vi "MainGUI.vi"() -> ()   [LabVIEW 2017]
uses:
  General/Controls/Queue Manager Actions.ctl
  General/Controls/MessagePacket.ctl
  General/Controls/QueueNames.ctl
  General/Controls/FGV Actions.ctl
  Hardware/Main Scan Processor Status.vi
  Hardware/Table Stage/Controls/Motion Translation Module Control.ctl
  General/Controls/Set Get Controls.ctl
  General/Controls/ScanType.ctl
  General/Controls/Translation Stage Types.ctl
  Hardware/Table Stage/Controls/Translation Stage Cluster.ctl
  General/Controls/System Parameters.ctl
panel:
  in  "Status":string
  in  "Quit":bool
  in  "Scan Type":T1
  in  "Acquire":bool
  in  "Control Panel":enum32{"Scan", "Config", "Manual Contorls"}(tab)
  in  "Y":u16=1 min=1 max=30 step=1
  in  "X":u16=1 min=1 max=30 step=1
  in  "Custom":bool
  in  "XY Image Resolution":T2(ring)
  in  "C Frame Ave.":u8=1 min=1 max=30 step=1
  in  "B Frame Ave.":u8=1 min=1 max=30 step=1
  in  "Display Channel":T3(ring)
  in  "Zoom Factor":u8(knob)=1 min=1 max=10 step=1 scale=1.0..10.0
  in  "Pixel Dwell Time":dbl[unit] min=0.0 max=0.01 step=1e-05
  in  "A Frame Ave.":u8=1 min=1 max=30 step=1
  in  "Pockel Cell Delay":dbl[unit] min=0.0 max=0.01 step=1e-05
  in  "Galvo Setting Time":dbl[unit] min=0.0 max=0.01 step=1e-05
  in  "Max Line Rate":dbl[unit] min=0.0 max=10.0 step=0.01
  in  "Objective EFL":dbl[unit] min=0.0 max=0.01 step=1e-05
  in  "Angular Mag.":dbl min=0.0 max=10.0 step=0.01
  in  "Center Galvos":bool
  out "Label Name":string[][](array[string])
  in  "System Parameters":T4={"Optical /HW Parameters"={"Focal Length [mm]"=1.0, "Scan Lens EFL[mm]"=0.0, "Tube Lens EFL[mm]"=0.0, "Galvo V Range (+/-)"=0.0, "Galvo Max Half Angle [Deg]"=0.0, "Max Galvo Range[%]"=0.0}, "Vibratome"={"Z Bottom [mm]"=0.0, "Pre Cut Dwell [s]"=0.0, "Blade Frequency [RPM]"=0, "Slice Speed [mm/s]"=0.0, "Post Cut Dwell [s]"=0.0, "Ramp Time [s]"=0.0, "Start X [mm]"=0.0, "Start Y [mm]"=0.0, "Slice Length [mm]"=0.0, "Slice Axis"=enum."X Axis", "Controller VISA Ref"="COM4"}, "Table Stages"={"X Stage"={"Position"=0.0, "Is.Enabled?"=FALSE, "Is.Connected?"=FALSE, "Device SN"="45876539", "AccelerationMaximum"=0.0, "VelocityMaximum"=0.0, "Acceleration"=0.0, "Velocity"=0.0, "waitTimeout (ms)"=0, "Model"=enum."None", "Is.Homed?"=FALSE}, "Y Stage"={"Position"=0.0, "Is.Enabled?"=FALSE, "Is.Connected?"=FALSE, "Device SN"="45876539", "AccelerationMaximum"=0.0, "VelocityMaximum"=0.0, "Acceleration"=0.0, "Velocity"=0.0, "waitTimeout (ms)"=0, "Model"=enum."None", "Is.Homed?"=FALSE}, "Z Stage"={"Position"=0.0, "Is.Enabled?"=FALSE, "Is.Connected?"=FALSE, "Device SN"="45876539", "AccelerationMaximum"=0.0, "VelocityMaximum"=0.0, "Acceleration"=0.0, "Velocity"=0.0, "waitTimeout (ms)"=0, "Model"=enum."None", "Is.Homed?"=FALSE}}, "Imaging Parameter"={"Pixel Dwell Time [ms]"=1.0, "XY Center [um]"={"X"=1.0, "Y"=1.0}, "Zoom Factor"=1.0, "Display Channel"=enum."Channel A", "XY Image Resolution"=enum."256 x 256", "Custom"=FALSE, "Custom Size"={"X"=1, "Y"=1}, "Averaging"={"A Frame Ave."=1, "B Frame Ave."=1, "C Frame Ave. "=1}}} {"Imaging Parameter"."Custom Size"."Y" min=1 max=30 step=1; "Imaging Parameter"."Custom Size"."X" min=1 max=30 step=1; "Imaging Parameter"."XY Center [um]"."Y" min=1.0 max=30.0 step=1.0; "Imaging Parameter"."XY Center [um]"."X" min=1.0 max=30.0 step=1.0; "Imaging Parameter"."Averaging"."C Frame Ave." min=1 max=30 step=1; "Imaging Parameter"."Averaging"."B Frame Ave." min=1 max=30 step=1; "Imaging Parameter"."Averaging"."A Frame Ave." min=1 max=30 step=1; "Imaging Parameter"."Zoom Factor" min=1.0 max=10.0 step=0.1 scale=1.0..30.0; "Imaging Parameter"."Pixel Dwell Time [ms]" min=0.0 max=10.0 step=0.01}
  out "Control Class ID":u32[](array[numeric])
  out "Image":T7(plugin-control)
  # "Imaging Controls"
  # "X"
  # "GENERAL SETTINGS"
  # "SOURCE SETTINGS"
  # "X"
  # "X"
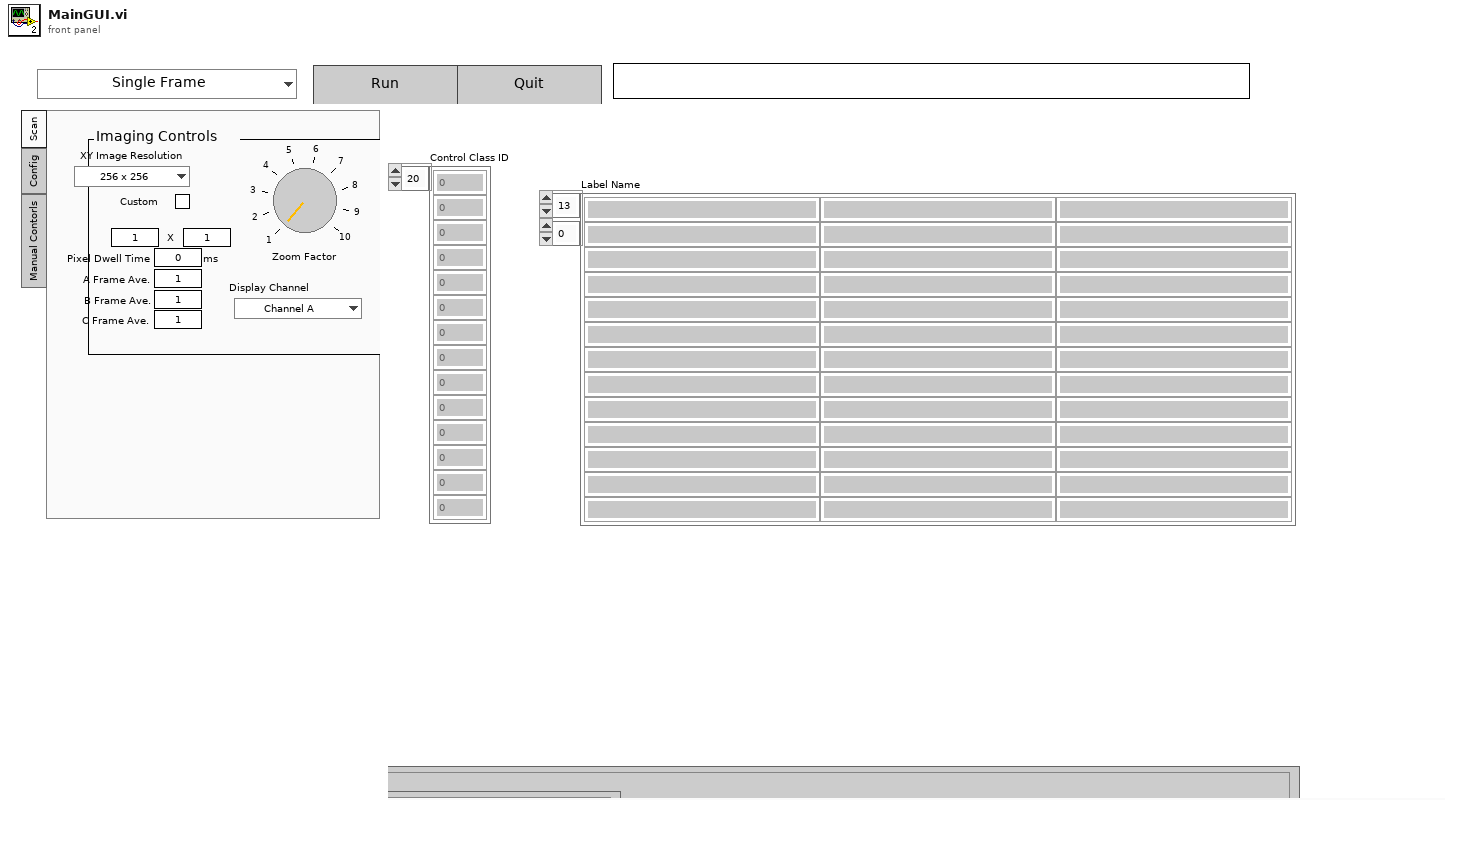
[diagram p1: front panel]
types:
  T1 = typedef "ScanType.ctl" = enum16{"Single Frame", "Continuous Frame", "ROI Line", "Vibratome", "Mosaic", "Mosaic + Slice"}
  T2 = enum16{"256 x 256", "512 x 512", "1024 x 1024", "2048 x 2048"}
  T3 = enum16{"Channel A", "Channel B", "Channel A and B"}
  T4 = typedef "System Parameters.ctl" = cluster{"Optical /HW Parameters":cluster{"Focal Length [mm]":dbl, "Scan Lens EFL[mm]":dbl, "Tube Lens EFL[mm]":dbl, "Galvo V Range (+/-)":dbl, "Galvo Max Half Angle [Deg]":dbl, "Max Galvo Range[%]":dbl}, "Vibratome":cluster{"Z Bottom [mm]":dbl, "Pre Cut Dwell [s]":dbl, "Blade Frequency [RPM]":u16, "Slice Speed [mm/s]":dbl, "Post Cut Dwell [s]":dbl, "Ramp Time [s]":dbl, "Start X [mm]":dbl, "Start Y [mm]":dbl, "Slice Length [mm]":dbl, "Slice Axis":enum16{"X Axis", "Y Axis", "Z Axis"}, "Controller VISA Ref":refnum<visa-resource-name>}, "Table Stages":cluster{"X Stage":T5, "Y Stage":T5, "Z Stage":T5}, "Imaging Parameter":cluster{"Pixel Dwell Time [ms]":dbl, "XY Center [um]":cluster{"X":dbl, "Y":dbl}, "Zoom Factor":dbl, "Display Channel":enum16{"Channel A", "Channel B", "Channel A and B"}, "XY Image Resolution":enum16{"32 x 32", "64 x 64", "128 x 128", "256 x 256", "512 x 512", "1024 x 1024", "2048 x 2048"}, "Custom":bool, "Custom Size":cluster{"X":u16, "Y":u16}, "Averaging":cluster{"A Frame Ave.":u8, "B Frame Ave.":u8, "C Frame Ave. ":u8}}}
  T5 = typedef "Translation Stage Cluster.ctl" = cluster{"Position":dbl, "Is.Enabled?":bool, "Is.Connected?":bool, "Device SN":string, "AccelerationMaximum":dbl, "VelocityMaximum":dbl, "Acceleration":dbl, "Velocity":dbl, "waitTimeout (ms)":i32, "Model":T6, "Is.Homed?":bool}
  T6 = typedef "Translation Stage Types.ctl" = enum16{"None", "Thorlabs LTS", "Thorlabs MLJ"}
  T7 = typedef "IMAQ Image.ctl" = refnum<image>
  T8 = typedef "QueueNames.ctl" = enum16{"Main GUI", "Main Scan Processor", "Main Display", "Main Table Stage GUI", "Main Table Stage Proc.", "Scan Engine", "Vibratome GUI", "Vibratome Processor", "Slice Engine"}
  T9 = typedef "Queue Manager Actions.ctl" = enum16{"Init", "Enqueue", "Enqueue All", "Preview Queue", "Dequeue", "Get Status", "Flush Queue", "Flush All Queues", "Release All Queues", "Release Queue", "Enqueue at Opposite End"}
  T10 = typedef "MessagePacket.ctl" = cluster{"Message":string, "Parameter":variant}
  T11 = typedef "FGV Actions.ctl" = enum16{"Init", "Set", "Get", "Clear"}
  T12 = enum16{"Set Configuration", "Get Configuration", "Enable Motor", "Disable Motor", "Get Status", "Open Session", "Close Session", "Set Limits", "Get Limits"}
  T13 = typedef "Set Get Controls.ctl" = enum16{"Set", "Get"}
  T14 = typedef "Motion Translation Module Control.ctl" = enum16{"Init", "Home", "Status", "Velocity/Accel", "Position", "Jog", "Stop", "Uninit", "Enable", "Disable"}
  T15 = cluster{"X Stage":T5, "Y Stage":T5, "Z Stage":T5}
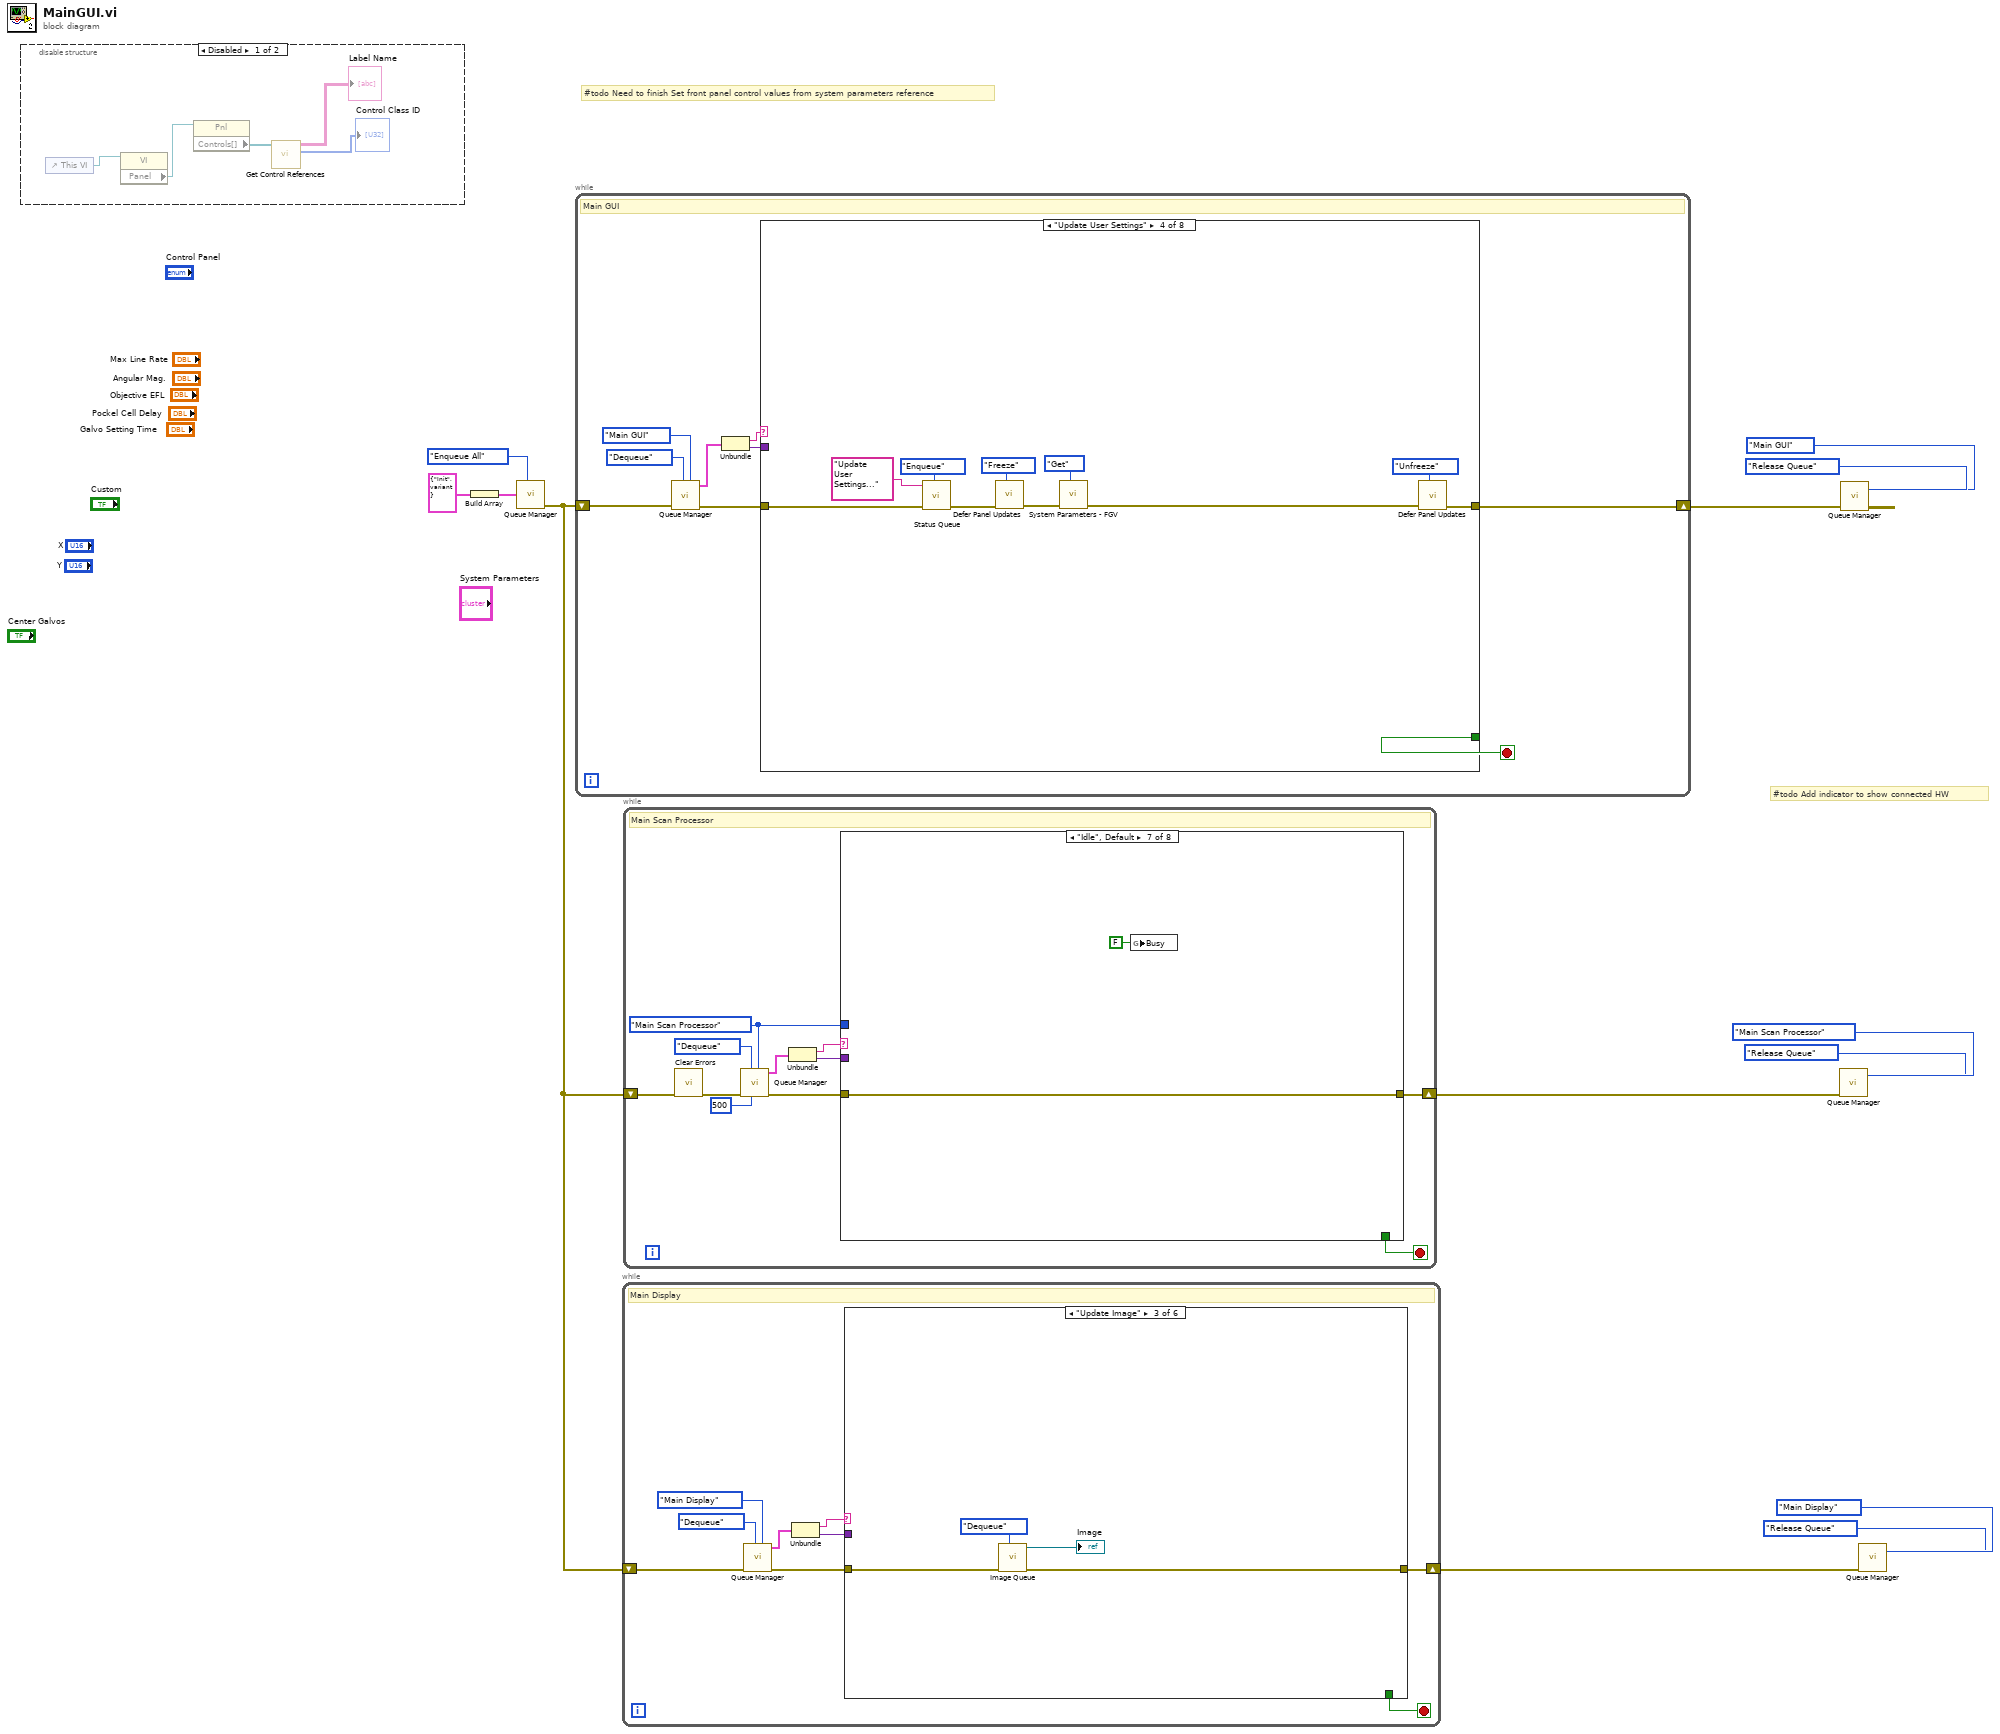
[diagram p0: block diagram]
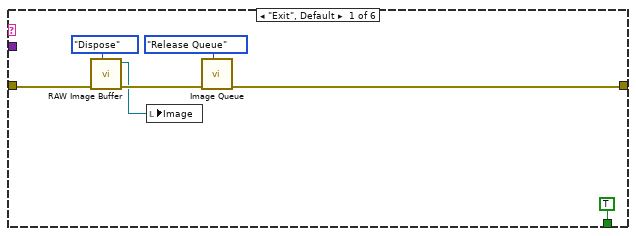
[diagram p3: hidden frame]
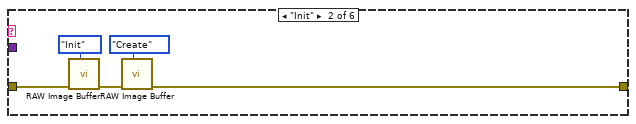
[diagram p4: hidden frame]
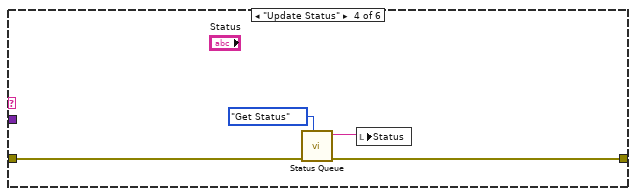
[diagram p5: hidden frame]
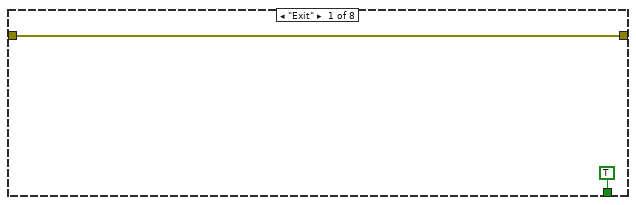
[diagram p8: hidden frame]
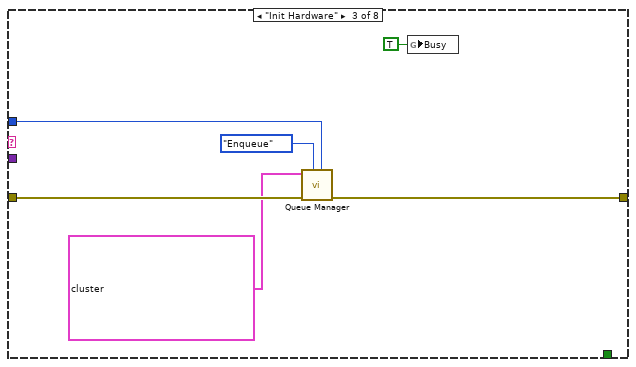
[diagram p10: hidden frame]
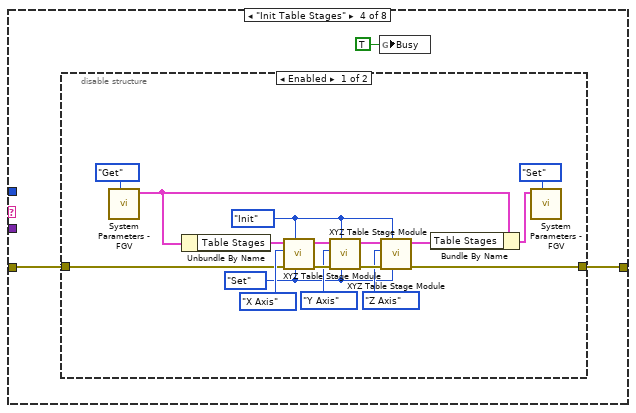
[diagram p11: hidden frame]
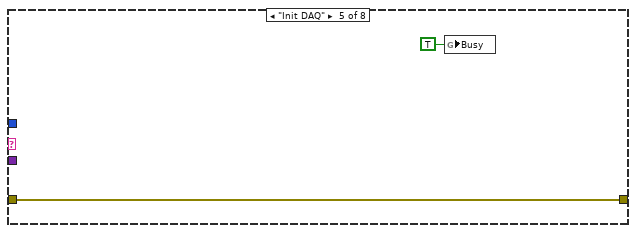
[diagram p13: hidden frame]
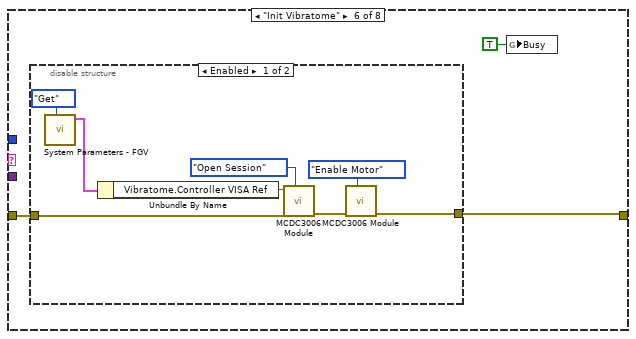
[diagram p14: hidden frame]
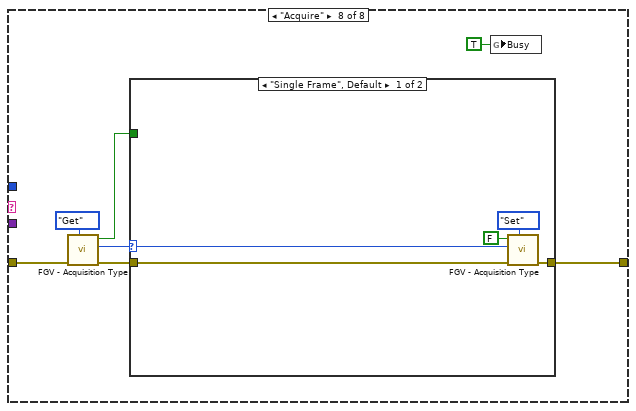
[diagram p16: hidden frame]
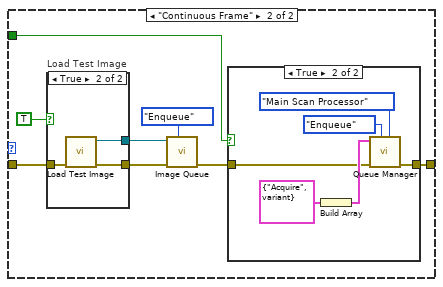
[diagram p17: hidden frame]
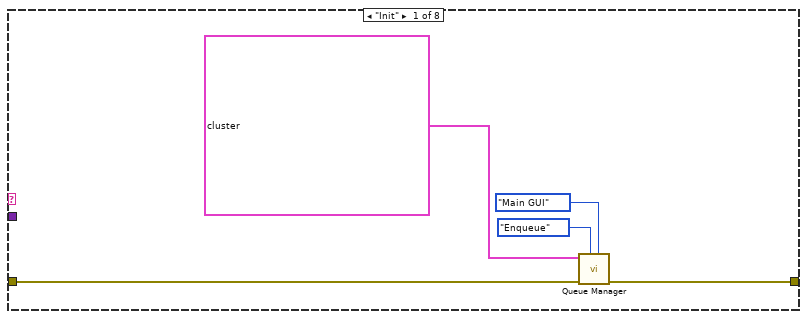
[diagram p20: hidden frame]
diagram:
  # "#todo Add indicator to show connected HW"
  # "#todo Need to finish Set front panel control values from system parameters reference"
  n1 = disable-structure shown="Disabled" {
    frame Disabled {
      n2 = control-ref of="This VI"() -> (w18:refnum<vi>)
      n3 = property class="VI"(reference=w18) -> ("Panel"=w17:refnum<vi>)  [unwired: 1 in, 2 out]
      n4 = property class="Pnl"(reference=w17) -> ("Controls[]"=w16:refnum<vi>[])  [unwired: 1 in, 2 out]
      n5 = call "Get Control References.vi"("Control References"=w16) -> ("Control Class ID"=→"Control Class ID":u32[], "Label Name"=→"Label Name":string[][])  [unwired: 8 in, 1 out]
    }
    frame Enabled {
    }
  }
  n6 = Build Array(T10 {"Message"="Init", "Parameter"=variant} ("Message Packet [In]")) -> (w11:T10[])
  n7 = call "Queue Manager.vi"("Action"=Queue_Manager_Actions."Enqueue All", "Message Packet Array"=w11) -> ("Error Out"=w1:errorcluster)  [unwired: 5 in, 4 out]
  n8 = while {
    shift-right: [w19] -> w10
    shift-left: w1 -> [w27]
    stop <- w22 stop-if-true
    # "Main GUI"
    n9 = call "Queue Manager.vi"("Queue Name"=QueueNames."Main GUI", "Action"=Queue_Manager_Actions."Dequeue", "Error In"=w27) -> ("Error Out"=w25:errorcluster, "Message Packet [Out]"=w24:T10)  [unwired: 4 in, 3 out]
    n10 = Unbundle(w24) -> ("Message"=w20:string, "Parameter"=w23:variant)
    n11 = case shown="\"Update User Settings\"" w20 {
      tunnel: w25 -> [w32 w49 w54 w80 w87 w101 w113 w227]
      tunnel: w23 -> [_ _ _ _ _ _ _ _]
      tunnel: [w31 w45 w50 w76 w83 w99 w114 w228] -> w19
      tunnel: [_ _ _ _ _ _ _ TRUE] -> w22
      frame "Init" {
        n12 = call "Queue Manager.vi"("Queue Name"=QueueNames."Main GUI", "Action"=Queue_Manager_Actions."Enqueue", "Error In"=w32, "Message Packet Array"=T10[] [{"Message"="Init Variables", "Parameter"=variant}, {"Message"="Set Front Panel", "Parameter"=variant}, {"Message"="Update User Settings", "Parameter"=variant}, {"Message"="Configure Hardware", "Parameter"=variant}, {"Message"="Wait for Complete", "Parameter"=variant}, {"Message"="Wait for User Input", "Parameter"=variant}]) -> ("Error Out"=w31:errorcluster)  [unwired: 3 in, 4 out]
      }
      frame "Init Variables" {
        n13 = control-ref of="This VI"() -> (w47:refnum<vi>)
        n14 = call "Status Queue.vi"("Action"=Queue_Manager_Actions."Enqueue", "Error In"=w49, "Status Message [In]"="Initializing Variables...") -> ("Error Out"=w44:errorcluster)  [unwired: 7 in, 1 out]
        n15 = call "Defer Panel Updates.vi"("Action"=enum16{"Init", "Freeze", "Unfreeze"}."Init", "Error In"=w44, "reference"=w47) -> ("Error Out"=w41:errorcluster)  [unwired: 8 in]
        n16 = call "System Parameters - FGV.vi"("Actions"=FGV_Actions."Init", "Error In"=w41) -> ("Error Out"=w36:errorcluster)  [unwired: 8 in, 1 out]
        n17 = call "Read Config from File.vi"("error in (no error)"=w36) -> ("error out"=w40:errorcluster, "System Parameters"=w37:T4)  [unwired: 9 in]
        n18 = call "System Parameters - FGV.vi"("Actions"=FGV_Actions."Set", "Error In"=w40, "System Parameters [In]"=w37) -> ("Error Out"=w39:errorcluster)  [unwired: 7 in, 1 out]
        n19 = call "FGV - Acquisition Type.vi"("Actions"=FGV_Actions."Init", "Error In"=w39) -> ("Error Out"=w45:errorcluster, "Scan Type [Out]"=w34:T1)  [unwired: 7 in, 1 out]
        n20 = local write "Scan Type"(w34) -> ()
        n21 = local write "Control Panel"(enum32{"Scan", "Config", "Manual Contorls"}."Scan" ("Control Panel")) -> ()
      }
      frame "Set Front Panel" {
        n22 = call "Status Queue.vi"("Action"=Queue_Manager_Actions."Enqueue", "Error In"=w54, "Status Message [In]"="Setting Front Panel Controls...") -> ("Error Out"=w55:errorcluster)  [unwired: 7 in, 1 out]
        n23 = call "Defer Panel Updates.vi"("Action"=enum16{"Init", "Freeze", "Unfreeze"}."Freeze", "Error In"=w55) -> ("Error Out"=w63:errorcluster)  [unwired: 9 in]
        n24 = call "FGV - Acquisition Type.vi"("Actions"=FGV_Actions."Get", "Error In"=w63) -> ("Error Out"=w60:errorcluster, "Scan Type [Out]"=w58:T1, "Status Out"=w59:bool)  [unwired: 7 in]
        n25 = case "Acquiring?" shown="False" w59 {
          tunnel: [w67 w72] -> w61
          tunnel: w60 -> [w68 w72]
          tunnel: w58 -> [w66 _]
          frame False {
            # "Non-Acquiring FP States"
            n26 = disable-structure shown="Enabled" {
              disable-tunnel: w68 -> [w71 _]
              disable-tunnel: [w70 _] -> w67
              disable-tunnel: w66 -> [w69 _]
              frame Enabled {
                n27 = call "Set Main GUI for Different Acquire States.vi"("Error In"=w71, "Scan Type"=w69) -> ("Error Out"=w70:errorcluster)  [unwired: 9 in]
              }
              frame Disabled {
              }
            }
          }
          frame True {
            # "Acquiring FP States"
          }
        }
        n28 = call "Defer Panel Updates.vi"("Action"=enum16{"Init", "Freeze", "Unfreeze"}."Unfreeze", "Error In"=w61) -> ("Error Out"=w51:errorcluster)  [unwired: 9 in]
        n29 = call "Status Queue.vi"("Action"=Queue_Manager_Actions."Enqueue", "Error In"=w51, "Status Message [In]"="Finished Setting Front Panel.") -> ("Error Out"=w50:errorcluster)  [unwired: 7 in, 1 out]
      }
      frame "Update User Settings" {
        n30 = call "Status Queue.vi"("Action"=Queue_Manager_Actions."Enqueue", "Error In"=w80, "Status Message [In]"="Update User Settings...") -> ("Error Out"=w78:errorcluster)  [unwired: 7 in, 1 out]
        n31 = call "Defer Panel Updates.vi"("Action"=enum16{"Init", "Freeze", "Unfreeze"}."Freeze", "Error In"=w78) -> ("Error Out"=w75:errorcluster)  [unwired: 9 in]
        n32 = call "System Parameters - FGV.vi"("Actions"=FGV_Actions."Get", "Error In"=w75) -> ("Error Out"=w73:errorcluster)  [unwired: 8 in, 1 out]
        n33 = call "Defer Panel Updates.vi"("Action"=enum16{"Init", "Freeze", "Unfreeze"}."Unfreeze", "Error In"=w73) -> ("Error Out"=w76:errorcluster)  [unwired: 9 in]
      }
      frame "Configure Hardware" {
        n34 = call "Status Queue.vi"("Action"=Queue_Manager_Actions."Enqueue", "Error In"=w87, "Status Message [In]"="Initializing Hardware...") -> ("Error Out"=w86:errorcluster)  [unwired: 7 in, 1 out]
        n35 = Build Array(T10 {"Message"="Init Hardware", "Parameter"=variant} ("Message Packet [In]")) -> (w84:T10[])
        n36 = call "Queue Manager.vi"("Queue Name"=QueueNames."Main Scan Processor", "Action"=Queue_Manager_Actions."Enqueue", "Error In"=w86, "Message Packet Array"=w84) -> ("Error Out"=w83:errorcluster)  [unwired: 3 in, 4 out]
      }
      frame "Wait for Complete" {
        n37 = call "TickTock.vi"("Error In"=w101) -> ("Error Out"=w97:errorcluster, "Current Time (Out)"=w96:timestamp)  [unwired: 8 in, 1 out]
        n38 = while {
          shift-right: [w104] -> w98
          shift-left: w97 -> [w112]
          tunnel: w96 -> [w111]
          tunnel: [w102] -> w95
          stop <- w103 stop-if-true
          n39 = call "Inline Wait.vi"("Error In"=w112, "milliseconds to wait"=u32 100) -> ("Error Out"=w108:errorcluster)  [unwired: 9 in]
          n40 = global read "Main Scan Processor Status.vi" "Busy"() -> (w106:bool)
          n41 = call "TickTock.vi"("Error In"=w108, "Current Time (In)"=w111) -> ("Error Out"=w104:errorcluster, "dt"=w110:dbl)  [unwired: 7 in, 1 out]
          n42 = Greater?(x=60000.0, y=w110) -> (0:w102:bool)
          n43 = Not(x=w106) -> (.not. x?=w105:bool)
          n44 = Or(x=w102, y=w105) -> (x .or. y?=w103:bool)
        }
        n45 = Select(t="Completed." ("Status Message [In]"), s=w95, f="Operation timed out." ("Status Message [In]")) -> (s? t:f=w92:string)
        n46 = call "Status Queue.vi"("Action"=Queue_Manager_Actions."Enqueue", "Error In"=w98, "Status Message [In]"=w92) -> ("Error Out"=w99:errorcluster)  [unwired: 7 in, 1 out]
      }
      frame "Wait for User Input" {
        n47 = event shown="[6] \"A Frame Ave.\", \"B Frame Ave.\", \"C Frame Ave.\": Value Change" {
          selector: _ -> [_ _ _ _ _ _ _ _ _]
          dyn-events: _ -> [_ _ _ _ _ _ _ _ _]
          timeout: _ -> [_ _ _ _ _ _ _ _ _]
          tunnel: [w115 w125 w131 w144 w162 w175 w190 w199 w214] -> w114
          tunnel: w113 -> [w115 w119 w133 w141 w160 w173 w188 w203 w216]
          event Timeout {
            n48 = event-data() -> ()  [unwired: 1 in, 3 out]
          }
          event "Quit": Value Change {
            n49 = event-data() -> ()  [unwired: 1 in, 1 out]
            n50 = call "Status Queue.vi"("Action"=Queue_Manager_Actions."Enqueue", "Error In"=w119, "Status Message [In]"="Exiting Software...") -> ("Error Out"=w118:errorcluster)  [unwired: 7 in, 1 out]
            n51 = call "Set Main GUI for Different Acquire States.vi"("Error In"=w118, "Scan Type"=ScanType."Single Frame" ("Scan Type [Out]")) -> ("Error Out"=w117:errorcluster)  [unwired: 9 in]
            n52 = Build Array(T10 {"Message"="Exit", "Parameter"=variant} ("Message Packet [In]")) -> (w122:T10[])
            n53 = call "Queue Manager.vi"("Action"=Queue_Manager_Actions."Enqueue All", "Error In"=w117, "Message Packet Array"=w122) -> ("Error Out"=w125:errorcluster)  [unwired: 4 in, 4 out]
          }
          event "Image": Value Change {
            w134 = 2 items=["No Event"=0, "Click Event"=1, "Draw Event"=2, "Size Event"=4, "Scroll Event"=5, "Double Click Event"=8]
            n54 = event-data() -> ("CtlRef"=w126:refnum<vi>)  [unwired: 1 in, 5 out]
            n55 = Build Array(w134) -> (w135:i32[])
            n56 = invoke class="ImageControl" method="Get Last Event"(reference=w126, error in=w133, "Which Events"=w135) -> (error out=w132:errorcluster)  [unwired: 5 in, 7 out]
            n57 = Build Array(T10 {"Message"="Wait for User Input", "Parameter"=variant} ("Message Packet [In]")) -> (w127:T10[])
            n58 = call "Queue Manager.vi"("Queue Name"=QueueNames."Main GUI", "Action"=Queue_Manager_Actions."Enqueue", "Error In"=w132, "Message Packet Array"=w127) -> ("Error Out"=w131:errorcluster)  [unwired: 3 in, 4 out]
          }
          event "XY Image Resolution": Value Change {
            n59 = event-data() -> ()  [unwired: 1 in, 1 out]
            n60 = Add(x="XY Image Resolution", y=5) -> (x+y=w151:i32)
            n61 = call "System Parameters - FGV.vi"("Actions"=FGV_Actions."Get", "Error In"=w141) -> ("Error Out"=w140:errorcluster, "System Parameters"=w138:T4)  [unwired: 8 in]
            n62 = Bundle By Name(cluster=w138, "Imaging Parameter.XY Image Resolution"="XY Image Resolution") -> (w137:T4)
            n63 = Power Of 2(x=w151) -> (2^x=w150:dbl)
            n64 = To Unsigned Word Integer(number=w150) -> (unsigned 16bit integer=w149:u16)
            n65 = local write "X"(w149) -> ()
            n66 = local write "Y"(w149) -> ()
            n67 = call "System Parameters - FGV.vi"("Actions"=FGV_Actions."Set", "Error In"=w140, "System Parameters [In]"=w137) -> ("Error Out"=w139:errorcluster)  [unwired: 7 in, 1 out]
            n68 = Build Array(T10 {"Message"="Wait for User Input", "Parameter"=variant} ("Message Packet [In]")) -> (w145:T10[])
            n69 = call "Queue Manager.vi"("Queue Name"=QueueNames."Main GUI", "Action"=Queue_Manager_Actions."Enqueue", "Error In"=w139, "Message Packet Array"=w145) -> ("Error Out"=w144:errorcluster)  [unwired: 3 in, 4 out]
          }
          event "Zoom Factor", "Pixel Dwell Time": Value Change {
            n70 = event-data() -> ()  [unwired: 1 in, 6 out]
            n71 = call "System Parameters - FGV.vi"("Actions"=FGV_Actions."Get", "Error In"=w160) -> ("Error Out"=w157:errorcluster, "System Parameters"=w156:T4)  [unwired: 8 in]
            n72 = Bundle By Name(cluster=w156, "Imaging Parameter.Zoom Factor"="Zoom Factor", "Pixel Dwell Time"="Pixel Dwell Time") -> (w155:T4)
            n73 = call "System Parameters - FGV.vi"("Actions"=FGV_Actions."Set", "Error In"=w157, "System Parameters [In]"=w155) -> ("Error Out"=w158:errorcluster)  [unwired: 7 in, 1 out]
            n74 = Build Array(T10 {"Message"="Wait for User Input", "Parameter"=variant} ("Message Packet [In]")) -> (w163:T10[])
            n75 = call "Queue Manager.vi"("Queue Name"=QueueNames."Main GUI", "Action"=Queue_Manager_Actions."Enqueue", "Error In"=w158, "Message Packet Array"=w163) -> ("Error Out"=w162:errorcluster)  [unwired: 3 in, 4 out]
          }
          event "Display Channel": Value Change {
            n76 = event-data() -> ()  [unwired: 1 in, 6 out]
            n77 = call "System Parameters - FGV.vi"("Actions"=FGV_Actions."Get", "Error In"=w173) -> ("Error Out"=w170:errorcluster, "System Parameters"=w169:T4)  [unwired: 8 in]
            n78 = Bundle By Name(cluster=w169, "Imaging Parameter.Display Channel"="Display Channel") -> (w168:T4)
            n79 = call "System Parameters - FGV.vi"("Actions"=FGV_Actions."Set", "Error In"=w170, "System Parameters [In]"=w168) -> ("Error Out"=w171:errorcluster)  [unwired: 7 in, 1 out]
            n80 = Build Array(T10 {"Message"="Wait for User Input", "Parameter"=variant} ("Message Packet [In]")) -> (w176:T10[])
            n81 = call "Queue Manager.vi"("Queue Name"=QueueNames."Main GUI", "Action"=Queue_Manager_Actions."Enqueue", "Error In"=w171, "Message Packet Array"=w176) -> ("Error Out"=w175:errorcluster)  [unwired: 3 in, 4 out]
          }
          event "A Frame Ave.", "B Frame Ave.", "C Frame Ave.": Value Change {
            n82 = event-data() -> ()  [unwired: 1 in, 6 out]
            n83 = call "System Parameters - FGV.vi"("Actions"=FGV_Actions."Get", "Error In"=w188) -> ("Error Out"=w185:errorcluster, "System Parameters"=w184:T4)  [unwired: 8 in]
            n84 = Bundle By Name(cluster=w184, "Imaging Parameter.Averaging.A Frame Ave."="A Frame Ave.", "Imaging Parameter.Averaging.B Frame Ave."="B Frame Ave.", "Imaging Parameter.Averaging.C Frame Ave."="C Frame Ave.") -> (w183:T4)
            n85 = call "System Parameters - FGV.vi"("Actions"=FGV_Actions."Set", "Error In"=w185, "System Parameters [In]"=w183) -> ("Error Out"=w186:errorcluster)  [unwired: 7 in, 1 out]
            n86 = Build Array(T10 {"Message"="Wait for User Input", "Parameter"=variant} ("Message Packet [In]")) -> (w191:T10[])
            n87 = call "Queue Manager.vi"("Queue Name"=QueueNames."Main GUI", "Action"=Queue_Manager_Actions."Enqueue", "Error In"=w186, "Message Packet Array"=w191) -> ("Error Out"=w190:errorcluster)  [unwired: 3 in, 4 out]
          }
          event Value Change {
            n88 = event-data() -> ()  [unwired: 1 in, 6 out]
            n89 = call "Queue Manager.vi"("Queue Name"=QueueNames."Main GUI", "Action"=Queue_Manager_Actions."Enqueue", "Error In"=w203, "Message Packet Array"=T10[] [{"Message"="Set Front Panel", "Parameter"=variant}, {"Message"="Wait for User Input", "Parameter"=variant}]) -> ("Error Out"=w199:errorcluster)  [unwired: 3 in, 4 out]
            n90 = call "FGV - Acquisition Type.vi"("Actions"=FGV_Actions."Get") -> ("Status Out"=w198:bool)  [unwired: 8 in, 2 out]
            n91 = call "FGV - Acquisition Type.vi"("Actions"=FGV_Actions."Set", "Scan Type [In]"="Scan Type", "Status In"=w198) -> ()  [unwired: 6 in, 3 out]
          }
          event "Acquire": Value Change {
            w213 = Queue_Manager_Actions."Enqueue" ("Action")
            n92 = event-data() -> ()  [unwired: 1 in, 6 out]
            n93 = call "FGV - Acquisition Type.vi"("Actions"=FGV_Actions."Get") -> ("Error Out"=w206:errorcluster, "Scan Type [Out]"=w204:T1)  [unwired: 8 in, 1 out]
            n94 = call "Queue Manager.vi"("Queue Name"=QueueNames."Main GUI", "Action"=w213, "Error In"=w216, "Message Packet Array"=T10[] [{"Message"="Wait for User Input", "Parameter"=variant}]) -> ("Error Out"=w215:errorcluster)  [unwired: 3 in, 4 out]
            n95 = call "FGV - Acquisition Type.vi"("Actions"=FGV_Actions."Get") -> ("Status Out"=w207:bool)  [unwired: 8 in, 2 out]
            n96 = Not(x=w207) -> (.not. x?=w208:bool)
            n97 = case "Start Acquisition?" shown="False" w207 {
              tunnel: w215 -> [w222 w223]
              tunnel: [w221 w223] -> w214
              tunnel: w213 -> [w220 _]
              frame False {
                # "Starts Acquisition if Current Acquisition Status is \"Off\""
                n98 = Build Array(T10 {"Message"="Acquire", "Parameter"=variant} ("Message Packet [In]")) -> (w217:T10[])
                n99 = call "Queue Manager.vi"("Queue Name"=QueueNames."Main Scan Processor", "Action"=w220, "Error In"=w222, "Message Packet Array"=w217) -> ("Error Out"=w221:errorcluster)  [unwired: 3 in, 4 out]
              }
              frame True {
                # "Stops Acquisition if Current Status is On"
              }
            }
            n100 = call "FGV - Acquisition Type.vi"("Actions"=FGV_Actions."Set", "Error In"=w206, "Scan Type [In]"=w204, "Status In"=w208) -> ()  [unwired: 5 in, 3 out]
          }
        }
      }
      frame "Exit", Default {
        n101 = call "System Parameters - FGV.vi"("Actions"=FGV_Actions."Get", "Error In"=w227) -> ("Error Out"=w226:errorcluster, "System Parameters"=w224:T4)  [unwired: 8 in]
        n102 = call "Write Config to File.vi"("error in (no error)"=w226, "System Parameters"=w224) -> ("error out"=w228:errorcluster)  [unwired: 9 in]
      }
    }
  }
  n103 = while {
    shift-right: [w231] -> w3
    shift-left: w1 -> [w236]
    stop <- w230 stop-if-true
    # "Main Display"
    n104 = call "Queue Manager.vi"("Queue Name"=QueueNames."Main Display", "Action"=Queue_Manager_Actions."Dequeue", "Error In"=w236) -> ("Error Out"=w235:errorcluster, "Message Packet [Out]"=w234:T10)  [unwired: 4 in, 3 out]
    n105 = Unbundle(w234) -> ("Message"=w233:string, "Parameter"=w232:variant)
    n106 = case shown="\"Update Image\"" w233 {
      tunnel: w235 -> [w243 w250 w254 w258 w259 w260]
      tunnel: w232 -> [_ _ _ _ _ _]
      tunnel: [w241 w246 w253 w257 w259 w260] -> w231
      tunnel: [TRUE _ _ _ _ _] -> w230
      frame "Exit", Default {
        n107 = call "RAW Image Buffer.vi"("Actions"=enum16{"Init", "Create", "Get", "Dispose"}."Dispose", "Error In"=w243) -> ("Error Out"=w242:errorcluster, "Image Out"=w239:T7)  [unwired: 8 in]
        n108 = local write "Image"(w239) -> ()
        n109 = call "Image Queue.vi"("Action"=Queue_Manager_Actions."Release Queue", "Error In"=w242) -> ("Error Out"=w241:errorcluster)  [unwired: 8 in, 1 out]
      }
      frame "Init" {
        n110 = call "RAW Image Buffer.vi"("Actions"=enum16{"Init", "Create", "Get", "Dispose"}."Init", "Error In"=w250) -> ("Error Out"=w249:errorcluster)  [unwired: 8 in, 1 out]
        n111 = call "RAW Image Buffer.vi"("Actions"=enum16{"Init", "Create", "Get", "Dispose"}."Create", "Error In"=w249) -> ("Error Out"=w246:errorcluster)  [unwired: 8 in, 1 out]
      }
      frame "Update Image" {
        n112 = call "Image Queue.vi"("Action"=Queue_Manager_Actions."Dequeue", "Error In"=w254) -> ("Error Out"=w253:errorcluster, "Image Out"=→"Image":T7)  [unwired: 8 in]
      }
      frame "Update Status" {
        n113 = call "Status Queue.vi"("Action"=Queue_Manager_Actions."Get Status", "Error In"=w258) -> ("Error Out"=w257:errorcluster, "Status Message [Out]"=w255:string)  [unwired: 8 in]
        n114 = local write "Status"(w255) -> ()
      }
      frame "Update Line Profile" {
      }
      frame "Idle" {
      }
    }
  }
  n115 = while {
    shift-right: [w265] -> w5
    shift-left: w1 -> [w270]
    stop <- w264 stop-if-true
    w263 = QueueNames."Main Scan Processor" ("Queue Name")
    # "Main Scan Processor"
    n116 = call <vilib>:"Clear Errors.vi"("error in (no error)"=w270) -> ("error out"=w261:errorcluster)  [unwired: 5 in, 1 out]
    n117 = call "Queue Manager.vi"("Queue Name"=w263, "timeout in ms (-1)"=500, "Action"=Queue_Manager_Actions."Dequeue", "Error In"=w261) -> ("Error Out"=w269:errorcluster, "Message Packet [Out]"=w268:T10)  [unwired: 3 in, 3 out]
    n118 = Unbundle(w268) -> ("Message"=w267:string, "Parameter"=w266:variant)
    n119 = case shown="\"Idle\", Default" w267 {
      tunnel: w269 -> [w272 w274 w280 w283 w303 w305 w317 w319]
      tunnel: w266 -> [_ _ _ _ _ _ _ _]
      tunnel: [w272 w274 w279 w282 w303 w304 w317 w324] -> w265
      tunnel: [TRUE _ _ _ _ _ _ _] -> w264
      tunnel: w263 -> [_ _ w278 _ _ _ _ _]
      frame "Exit" {
      }
      frame "Init" {
      }
      frame "Init Hardware" {
        n120 = call "Queue Manager.vi"("Queue Name"=w278, "Action"=Queue_Manager_Actions."Enqueue", "Error In"=w280, "Message Packet Array"=T10[] [{"Message"="Init Table Stages", "Parameter"=variant}, {"Message"="Init DAQ", "Parameter"=variant}, {"Message"="Init Vibratome", "Parameter"=variant}, {"Message"="Idle", "Parameter"=variant}]) -> ("Error Out"=w279:errorcluster)  [unwired: 3 in, 4 out]
        n121 = global write "Main Scan Processor Status.vi" "Busy"(TRUE ("Busy")) -> ()
      }
      frame "Init Table Stages" {
        n122 = disable-structure shown="Enabled" {
          disable-tunnel: w283 -> [w291 w301]
          disable-tunnel: [w290 w301] -> w282
          frame Enabled {
            w292 = Set_Get_Controls."Set" ("Set/Get")
            w298 = Motion_Translation_Module_Control."Init" ("Action")
            n123 = call "System Parameters - FGV.vi"("Actions"=FGV_Actions."Get") -> ("System Parameters"=w286:T4)  [unwired: 9 in, 1 out]
            n124 = Unbundle By Name(w286) -> ("Table Stages"=w288:T15)
            n125 = call "XYZ Table Stage Module.vi"("Set/Get"=w292, "Action"=w298, "Error In"=w291, "Axis"=enum16{"X Axis", "Y Axis", "Z Axis"}."X Axis", "Table Stages"=w288) -> ("Error Out"=w300:errorcluster, "Table Stages Out"=w297:T15)  [unwired: 5 in]
            n126 = call "XYZ Table Stage Module.vi"("Set/Get"=w292, "Action"=w298, "Error In"=w300, "Axis"=enum16{"X Axis", "Y Axis", "Z Axis"}."Y Axis", "Table Stages"=w297) -> ("Error Out"=w299:errorcluster, "Table Stages Out"=w296:T15)  [unwired: 5 in]
            n127 = call "XYZ Table Stage Module.vi"("Set/Get"=w292, "Action"=w298, "Error In"=w299, "Axis"=enum16{"X Axis", "Y Axis", "Z Axis"}."Z Axis", "Table Stages"=w296) -> ("Error Out"=w290:errorcluster, "Table Stages Out"=w284:T15)  [unwired: 5 in]
            n128 = Bundle By Name(cluster=w286, "Table Stages"=w284) -> (w285:T4)
            n129 = call "System Parameters - FGV.vi"("Actions"=FGV_Actions."Set", "System Parameters [In]"=w285) -> ()  [unwired: 8 in, 2 out]
          }
          frame Disabled {
          }
        }
        n130 = global write "Main Scan Processor Status.vi" "Busy"(TRUE ("Busy")) -> ()
      }
      frame "Init DAQ" {
        n131 = global write "Main Scan Processor Status.vi" "Busy"(TRUE ("Busy")) -> ()
      }
      frame "Init Vibratome" {
        n132 = disable-structure shown="Enabled" {
          disable-tunnel: w305 -> [w311 w315]
          disable-tunnel: [w310 w315] -> w304
          frame Enabled {
            n133 = call "System Parameters - FGV.vi"("Actions"=FGV_Actions."Get") -> ("System Parameters"=w308:T4)  [unwired: 9 in, 1 out]
            n134 = Unbundle By Name(w308) -> ("Vibratome.Controller VISA Ref"=w307:refnum<visa-resource-name>)
            n135 = call "MCDC3006 Module.vi"("Actions"=T12."Open Session", "Error In"=w311, "VISA resource name"=w307) -> ("Error Out"=w313:errorcluster)  [unwired: 4 in, 4 out]
            n136 = call "MCDC3006 Module.vi"("Actions"=T12."Enable Motor", "Error In"=w313) -> ("Error Out"=w310:errorcluster)  [unwired: 5 in, 4 out]
          }
          frame Disabled {
          }
        }
        n137 = global write "Main Scan Processor Status.vi" "Busy"(TRUE ("Busy")) -> ()
      }
      frame "Idle", Default {
        n138 = global write "Main Scan Processor Status.vi" "Busy"(FALSE ("Busy")) -> ()
      }
      frame "Acquire" {
        n139 = call "FGV - Acquisition Type.vi"("Actions"=FGV_Actions."Get", "Error In"=w319) -> ("Error Out"=w320:errorcluster, "Scan Type [Out]"=w322:T1, "Status Out"=w321:bool)  [unwired: 7 in]
        n140 = case shown="\"Single Frame\", Default" w322 {
          selector: w322 -> [w326 _]
          tunnel: w320 -> [w327 w337]
          tunnel: [w328 w336] -> w324
          tunnel: w321 -> [_ w331]
          frame "Single Frame", Default {
            n141 = call "FGV - Acquisition Type.vi"("Actions"=FGV_Actions."Set", "Error In"=w327, "Scan Type [In]"=w326, "Status In"=FALSE) -> ("Error Out"=w328:errorcluster)  [unwired: 5 in, 2 out]
          }
          frame "Continuous Frame" {
            n142 = case "Load Test Image" shown="True" TRUE {
              tunnel: w337 -> [w345 w348]
              tunnel: [w345 w347] -> w334
              tunnel: [_ w346] -> w332
              frame False {
              }
              frame True {
                n143 = call "Load Test Image.vi"("Error In"=w348) -> ("Error Out"=w347:errorcluster, "Image"=w346:T7)  [unwired: 9 in]
              }
            }
            n144 = call "Image Queue.vi"("Action"=Queue_Manager_Actions."Enqueue", "Error In"=w334, "Image In"=w332) -> ("Error Out"=w330:errorcluster)  [unwired: 7 in, 1 out]
            n145 = case shown="True" w331 {
              tunnel: [w338 w344] -> w336
              tunnel: w330 -> [w338 w339]
              frame False {
              }
              frame True {
                n146 = Build Array(T10 {"Message"="Acquire", "Parameter"=variant} ("Message Packet [In]")) -> (w340:T10[])
                n147 = call "Queue Manager.vi"("Queue Name"=QueueNames."Main Scan Processor", "Action"=Queue_Manager_Actions."Enqueue", "Error In"=w339, "Message Packet Array"=w340) -> ("Error Out"=w344:errorcluster)  [unwired: 3 in, 4 out]
              }
            }
          }
        }
        n148 = global write "Main Scan Processor Status.vi" "Busy"(TRUE ("Busy")) -> ()
      }
    }
  }
  n149 = call "Queue Manager.vi"("Queue Name"=QueueNames."Main Scan Processor", "Action"=Queue_Manager_Actions."Release Queue", "Error In"=w5) -> ()  [unwired: 4 in, 5 out]
  n150 = call "Queue Manager.vi"("Queue Name"=QueueNames."Main GUI", "Action"=Queue_Manager_Actions."Release Queue", "Error In"=w10) -> ()  [unwired: 4 in, 5 out]
  n151 = call "Queue Manager.vi"("Queue Name"=QueueNames."Main Display", "Action"=Queue_Manager_Actions."Release Queue", "Error In"=w3) -> ()  [unwired: 4 in, 5 out]
